vi "extract_carriers.vi"(0 "Carrier amplitudes":T14 format="%#_3p", 2 "Config":T15={"IO params"={"Conversion"={"Rate"=4.0, "Num cards"=2, "Out channels"=4}, "Carriers"={"Phase shift"=180.0, "Levels"=[[0.8, 0.8, 0.8], [0.03, 0.03, 0.03]], "Delay samples"=73.15}, "TCP"={"Host"="192.168.1.15", "Port"=6666, "Buffering"=6, "Timeout"=6}, "Input channel sign"=[1, 1, 1]}, "High rate STFT"={"Win param"=101.5, "Window type"=61, "Win order"=2, "DFT size"=64, "Channels"=[7], "Oversample"=64}, "Low rate STFT"={"Win param"=120.0, "Window type"=61, "Win order"=8, "DFT size"=64, "Channels"=[7], "Oversample"=64}, "Filtering "=[]} {"Filtering"."Distortion"."Limit" format="%#_3p"; "Filtering"."Distortion"."LF cut" format="%#_3p"; "Filtering"."Kalman"."Measure noise" format="%#_3p"; "Filtering"."Kalman"."Process noise" format="%#_3p"; "Filtering"."Hum"."Limit" format="%#_3p"; "Filtering"."Hum"."Frequency" format="%#_4p"; "Low rate STFT"."Oversample" min=1 step=1; "Low rate STFT"."Channels" min=0 step=1; "Low rate STFT"."DFT size" min=1 step=1; "Low rate STFT"."Window type" items=["Rectangle"=0, "Hanning"=1, "Hamming"=2, "Blackman-Harris"=3, "Exact Blackman"=4, "Blackman"=5, "Flat Top"=6, "4 Term B-Harris "=7, "7 Term B-Harris"=8, "Low Sidelobe"=9, "Blackman Nuttall"=11, "Triangle"=30, "Bartlett-Hanning"=31, "Bohman"=32, "Parzen"=33, "Welch"=34, "Kaiser"=60, "Dolph-Chebyshev"=61, "Gaussian"=62]; "High rate STFT"."Oversample" min=1 step=1; "High rate STFT"."Channels" min=0 step=1; "High rate STFT"."DFT size" min=1 step=1; "High rate STFT"."Window type" items=["Rectangle"=0, "Hanning"=1, "Hamming"=2, "Blackman-Harris"=3, "Exact Blackman"=4, "Blackman"=5, "Flat Top"=6, "4 Term B-Harris "=7, "7 Term B-Harris"=8, "Low Sidelobe"=9, "Blackman Nuttall"=11, "Triangle"=30, "Bartlett-Hanning"=31, "Bohman"=32, "Parzen"=33, "Welch"=34, "Kaiser"=60, "Dolph-Chebyshev"=61, "Gaussian"=62]; "IO params"."Input channel sign" min=-1 max=1 step=1; "IO params"."Carriers"."Levels" min=0.0 step=0.1; "IO params"."Conversion"."Rate" format="%#_8g"}, 3 "Modulation info":T21={"Fs full"=0.0, "Fs high"=0.0, "Fs low"=0.0, "Read size"=0, "FFT size low"=5000, "df low"=5000.0, "High carriers"=[], "Low carriers"=[], "Hi channels at low"=[7]} {"Hi channels at low" min=0 step=1; "Low carriers" format="%#_6p"; "High carriers" format="%#_6p"}, 4 "Demodulated signal":T1 format="%#_3p", 5 "Ref carrier amplitudes":T14 format="%#_3p", 7 "Display options":T2={"Display card"=0, "Signal"=enum."Raw data", "Source axis"=enum."X", "Sensor axis"=enum."X", "Spectrum parameters"={"Window"=enum."7 Term B-Harris", "FFT blocking"=enum."1", "Averaging"=5.0, "Order"=2}, "AC/DC"=FALSE, "Amplitude/Phase"=FALSE, "Levels selectors"=[], "Map selector"=enum."fire", "Restart Averaging"=FALSE, "Noise ref"=FALSE} {"Spectrum parameters"."Order" min=1 max=100; "Spectrum parameters"."Averaging" min=0.0 max=1000.0 step=1.0}, 8 "Level selector":T6, 9 "Spectrum":waveform(cdb)[](array[waveform]), 10 "Trace info":T11, 11 "Noise floor":dbl[][](array[numeric]) format="%#_6p") -> (14 "Levels":dbl[][](array[numeric]) format="%.3f")   [LabVIEW 2026]
uses:
  processing/modulation_info.ctl
  processing/ilemt_config.ctl
  system/IO_params.ctl
  processing/stft_params.ctl
  <vilib>/Analysis/4window.llb/windowTd.ctl
  processing/filter_params.ctl
  processing/detrend_mode.ctl
  processing/carrier_amplitudes.ctl
  levels_selector.ctl
  Level selector 1.ctl
  Level selector 4.ctl
  Level selector 3.ctl
  Level selector 2.ctl
  trace_info.ctl
  trace_channel.ctl
  main/ilemt_status.ctl
  display_options.ctl
  display_source.ctl
  axis_name.ctl
  spectrum_parameters.ctl
  processing/card_high_carrier_amplitudes.ctl
  processing/coupling_matrix.ctl
  <vilib>/Analysis/NI_AALPro.lvlib
panel:
  # "This VI generates user-friendly output arrays for the carrier levels and noise floor display."
  # "Complex demodulated signal, from get_display_data.  This is used to implement the \"Trace display\" source."
  # "High"
  # "Low"
  # "X"
  # "Y"
  # "Z"
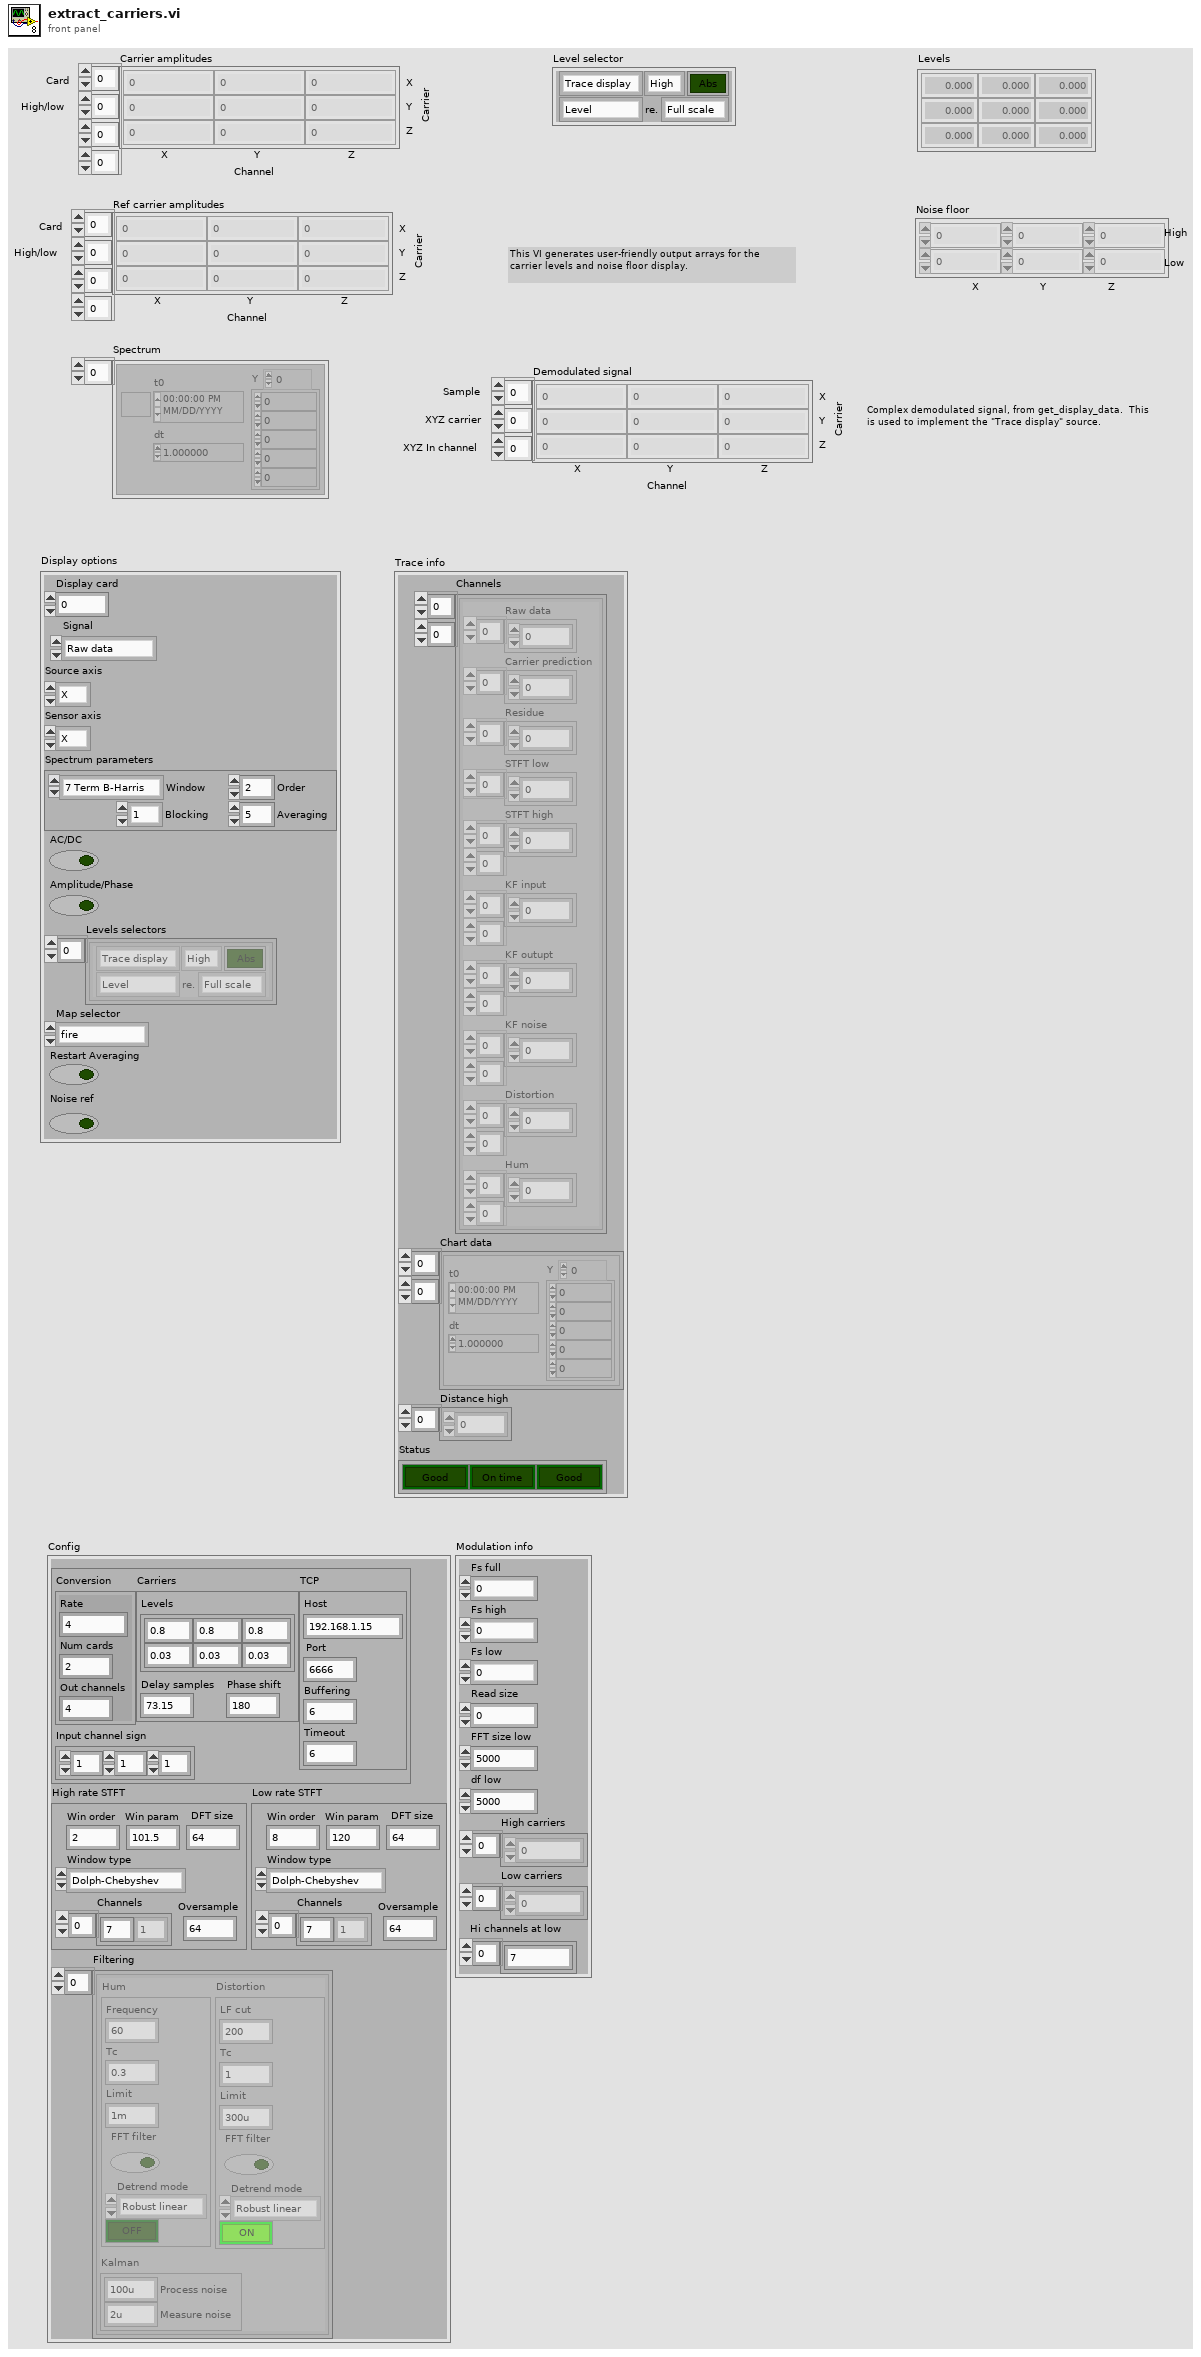
[diagram p1: front panel]
types:
  T1 = typedef "card_high_carrier_amplitudes.ctl" = cdb[][][]
  T2 = typedef "display_options.ctl" = cluster{"Display card":i32, "Signal":T3, "Source axis":T4, "Sensor axis":T4, "Spectrum parameters":T5, "AC/DC":bool, "Amplitude/Phase":bool, "Levels selectors":T6[], "Map selector":enum16{"fire", "rainbow", "grey", "inverse grey", "ice", "original"}, "Restart Averaging":bool, "Noise ref":bool}
  T3 = typedef "display_source.ctl" = enum16{"Raw data", "Carrier predict", "Residue", "STFT low", "STFT high", "KF input", "KF output", "KF noise", "Distortion", "Hum", "Distance high", "Chart high", "Chart low"}
  T4 = typedef "axis_name.ctl" = enum16{"X", "Y", "Z"}
  T5 = typedef "spectrum_parameters.ctl" = cluster{"Window":enum16{"None ", "Hanning", "Hamming", "Blackman-Harris", "Exact Blackman", "Blackman", "Flat Top", "4 Term B-Harris ", "7 Term B-Harris", "Low Sidelobe"}, "FFT blocking":enum16{"1", "2", "4", "8"}, "Averaging":dbl, "Order":u32}
  T6 = typedef "levels_selector.ctl" = cluster{"Signal source":T7, "Mode":T8, "re.":T9, "High/low":T10, "Sense":bool}
  T7 = typedef "Level selector 1.ctl" = enum16{"Trace display", "Carrier levels", "Ref levels"}
  T8 = typedef "Level selector 4.ctl" = enum16{"Level", "dB", "Phase", "Mismatch"}
  T9 = typedef "Level selector 3.ctl" = enum16{"Full scale", "Carrier", "Ref level", "Noise"}
  T10 = typedef "Level selector 2.ctl" = enum16{"High", "Low"}
  T11 = typedef "trace_info.ctl" = cluster{"Channels":T12[][], "Chart data":waveform(dbl)[][], "Distance high":dbl[], "Status":T13}
  T12 = typedef "trace_channel.ctl" = cluster{"Raw data":dbl[], "Carrier prediction":dbl[], "Residue":dbl[], "STFT low":cdb[], "STFT high":cdb[][], "KF input":cdb[][], "KF outupt":cdb[][], "KF noise":dbl[][], "Distortion":cdb[][], "Hum":cdb[][]}
  T13 = typedef "ilemt_status.ctl" = cluster{"NaN":bool, "Backlog":bool, "Clipping":bool}
  T14 = typedef "carrier_amplitudes.ctl" = cdb[][][][]
  T15 = typedef "ilemt_config.ctl" = cluster{"IO params":T16, "High rate STFT":T17, "Low rate STFT":T17, "Filtering ":T19[]}
  T16 = typedef "IO_params.ctl" = cluster{"Conversion":cluster{"Rate":dbl, "Num cards":u32, "Out channels":u32}, "Carriers":cluster{"Phase shift":dbl, "Levels":dbl[][], "Delay samples":dbl}, "TCP":cluster{"Host":string, "Port":i32, "Buffering":u32, "Timeout":u32}, "Input channel sign":i32[]}
  T17 = typedef "stft_params.ctl" = cluster{"Win param":dbl, "Window type":T18, "Win order":i32, "DFT size":i32, "Channels":i32[], "Oversample":i32}
  T18 = typedef "NI_AALPro.lvlib/windowTd.ctl" = u32
  T19 = typedef "filter_params.ctl" = cluster{"Hum":cluster{"Frequency":dbl, "Tc":dbl, "Limit":dbl, "FFT filter":bool, "Detrend mode":T20, "Enable":bool}, "Kalman":cluster{"Process noise":dbl, "Measure noise":dbl}, "Distortion":cluster{"LF cut":dbl, "Tc":dbl, "Limit":dbl, "FFT filter":bool, "Detrend mode":T20, "Enable":bool}}
  T20 = typedef "detrend_mode.ctl" = enum16{"Zero mean", "Linear", "Robust linear"}
  T21 = typedef "modulation_info.ctl" = cluster{"Fs full":dbl, "Fs high":dbl, "Fs low":dbl, "Read size":i32, "FFT size low":i32, "df low":dbl, "High carriers":dbl[], "Low carriers":dbl[], "Hi channels at low":i32[]}
  T22 = typedef "coupling_matrix.ctl" = cdb[][]
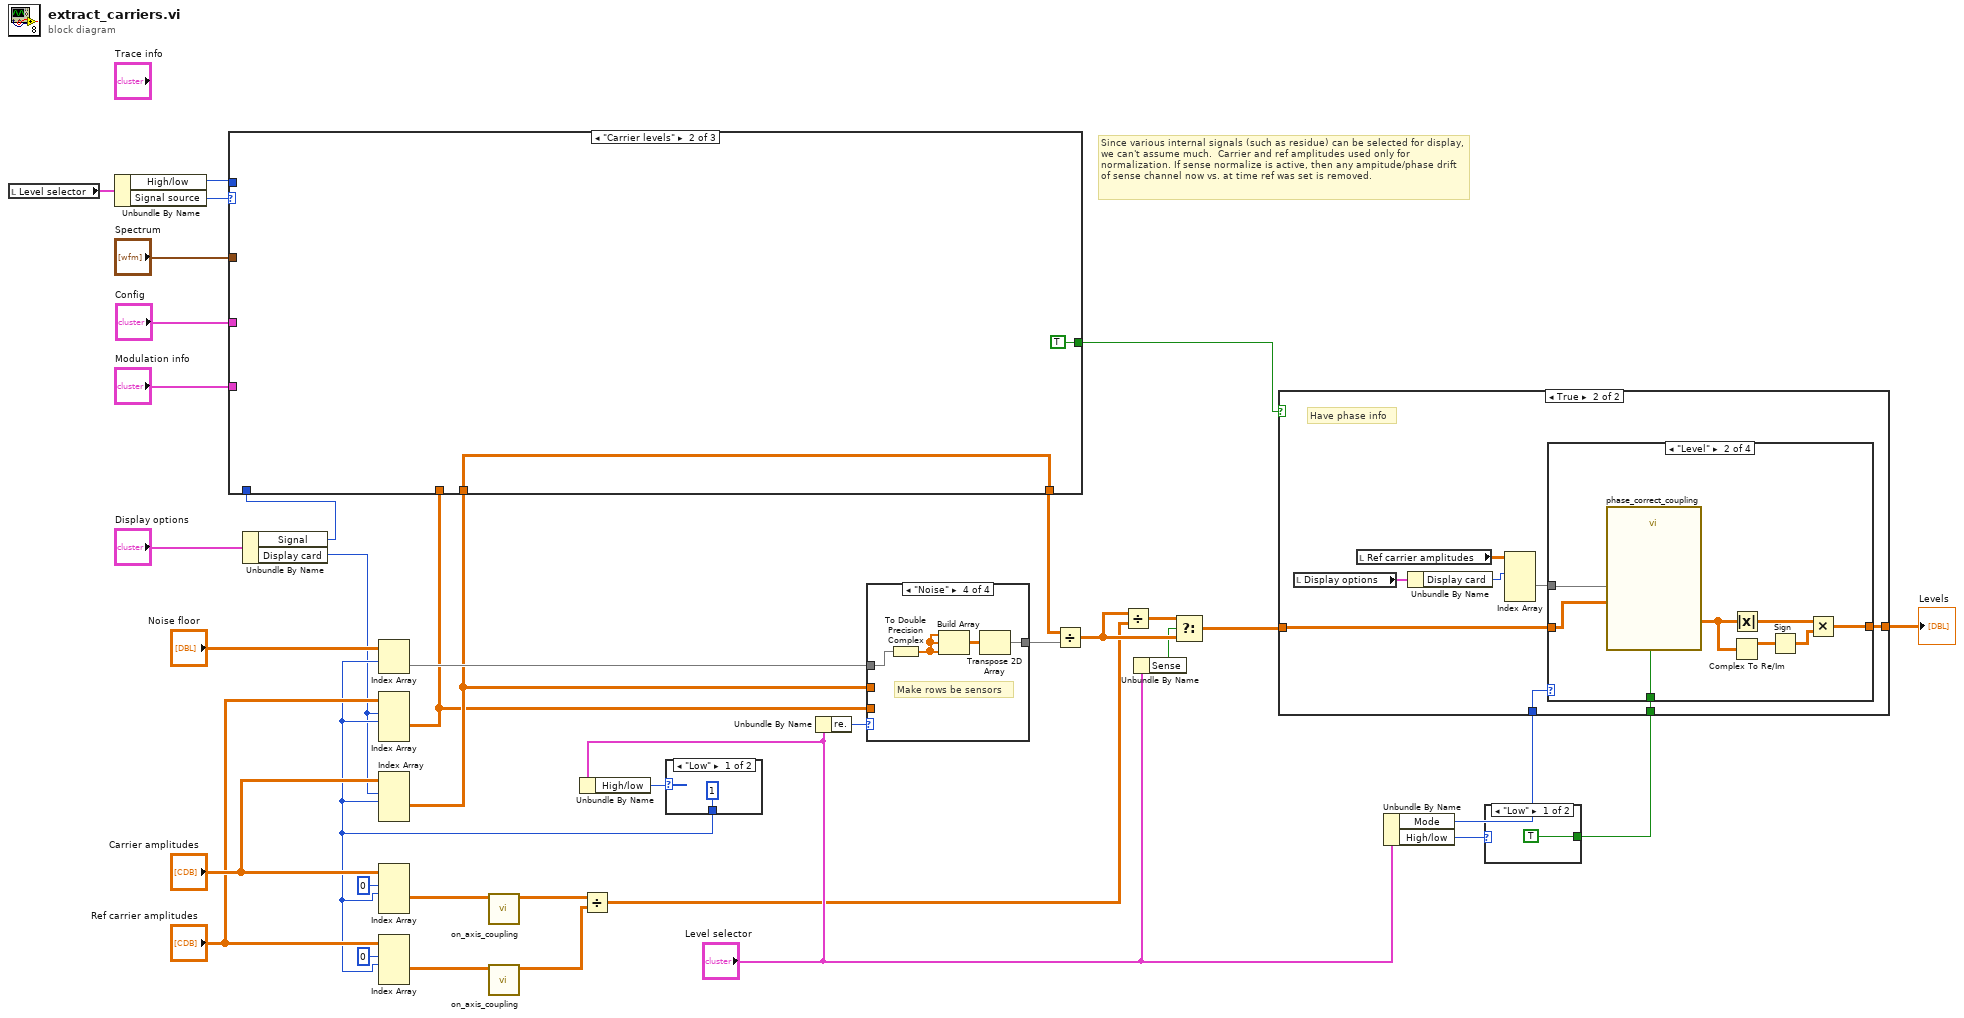
[diagram p0: block diagram]
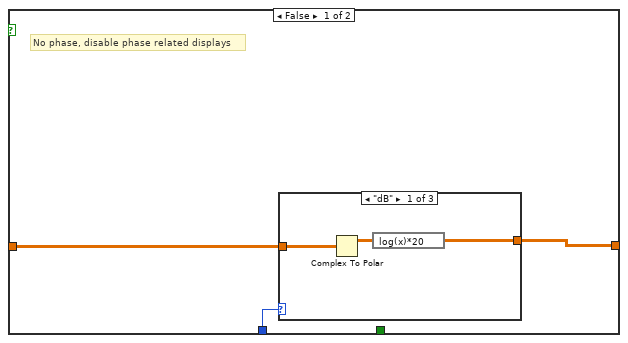
[diagram p2: hidden frame]
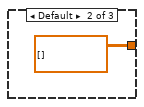
[diagram p3: hidden frame]
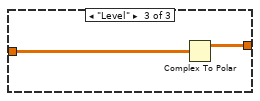
[diagram p4: hidden frame]
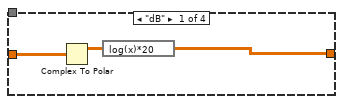
[diagram p5: hidden frame]
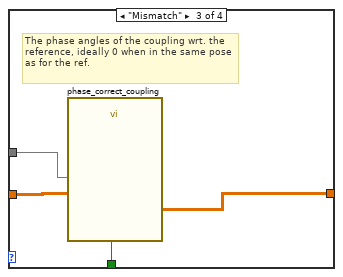
[diagram p6: hidden frame]
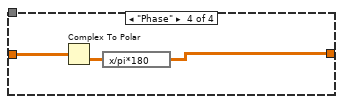
[diagram p7: hidden frame]
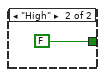
[diagram p8: hidden frame]
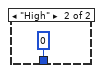
[diagram p9: hidden frame]
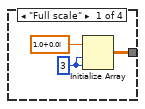
[diagram p10: hidden frame]
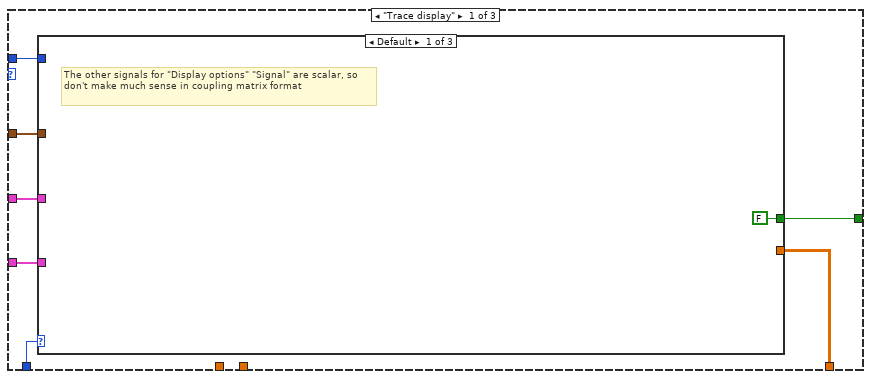
[diagram p13: hidden frame]
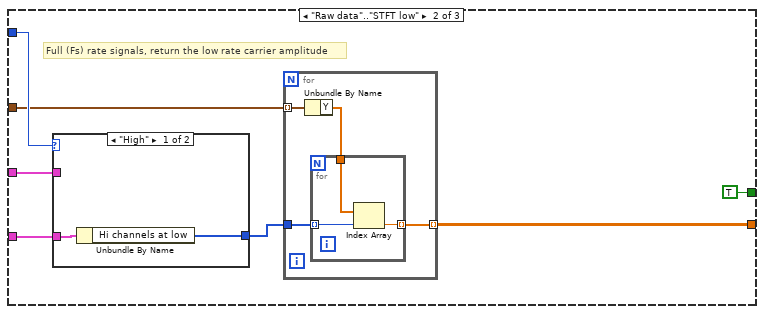
[diagram p14: hidden frame]
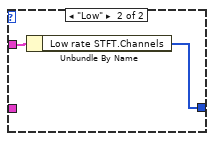
[diagram p15: hidden frame]
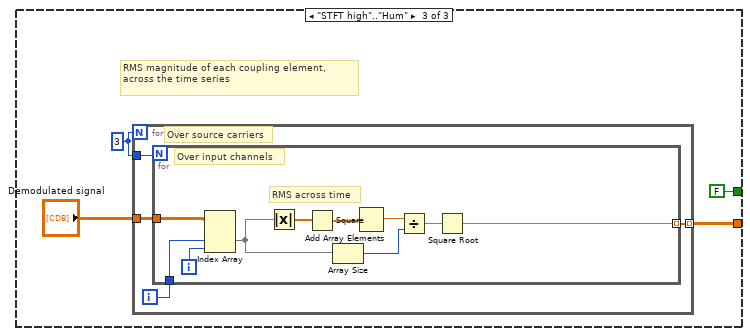
[diagram p16: hidden frame]
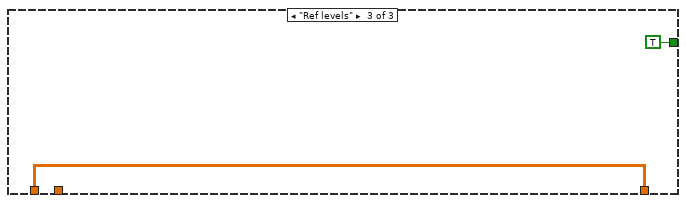
[diagram p17: hidden frame]
diagram:
  # "Since various internal signals (such as residue) can be selected for display, we can't assume much.  Carrier and ref amplitudes used only for normalization. If sense normalize is active, then any ampitude/phase drift of sense channel now vs. at time ref was set is removed."
  n1 = local read "Level selector"() -> (w25:T6)
  n2 = Unbundle By Name(w25) -> ("High/low"=w36:T10, "Signal source"=w37:T7)
  n3 = Unbundle By Name("Display options") -> ("Signal"=w7:T3, "Display card"=w3:i32)
  n4 = Unbundle By Name("Level selector") -> ("High/low"=w34:T10)
  n5 = case shown="\"Low\"" w34 {
    tunnel: [1 0] -> w11
    frame "Low" {
    }
    frame "High" {
    }
  }
  n6 = Index Array(array="Noise floor", index (row)=w11) -> (element=w23:dbl[])  [unwired: 1 in]
  n7 = Index Array(array="Ref carrier amplitudes", index (dim 0)=w3, index (dim 1)=w11) -> (element=w21:cdb[][])  [unwired: 2 in]
  n8 = Index Array(array="Carrier amplitudes", index (dim 0)=w3, index (dim 1)=w11) -> (element=w22:cdb[][])  [unwired: 2 in]
  n9 = case shown="\"Carrier levels\"" w37 {
    tunnel: [w45 w85 w87] -> w33
    tunnel: w36 -> [w46 _ _]
    tunnel: w22 -> [_ w85 _]
    tunnel: w21 -> [_ _ w87]
    tunnel: w7 -> [w44 _ _]
    tunnel: "Modulation info" -> [w43 _ _]
    tunnel: "Spectrum" -> [w42 _ _]
    tunnel: "Config" -> [w41 _ _]
    tunnel: [w40 TRUE TRUE] -> w1
    frame "Trace display" {
      n10 = case shown="Default" w44 {
        tunnel: w46 -> [_ w54 _]
        tunnel: [_ w53 w69] -> w45
        tunnel: w43 -> [_ w51 _]
        tunnel: w42 -> [_ w50 _]
        tunnel: w41 -> [_ w49 _]
        tunnel: [FALSE TRUE FALSE] -> w40
        frame Default {
          # "The other signals for \"Display options\" \"Signal\" are scalar, so don't make much sense in coupling matrix format"
        }
        frame "Raw data".."STFT low" {
          # "Full (Fs) rate signals, return the low rate carrier amplitude"
          n11 = case shown="\"High\"" w54 {
            tunnel: [w62 w64] -> w52
            tunnel: w49 -> [_ w65]
            tunnel: w51 -> [w63 _]
            frame "High" {
              n12 = Unbundle By Name(w63) -> ("Hi channels at low"=w62:i32[])
            }
            frame "Low" {
              n13 = Unbundle By Name(w65) -> ("Low rate STFT.Channels"=w64:i32[])
            }
          }
          n14 = for {
            tunnel: w50 -> [w56] mode=indexing
            tunnel: w52 -> [w58]
            tunnel: [w57] -> w53 mode=indexing
            n15 = Unbundle By Name(w56) -> ("Y"=w55:cdb[])
            n16 = for {
              tunnel: w58 -> [w59] mode=indexing
              tunnel: w55 -> [w61]
              tunnel: [w60] -> w57 mode=indexing
              n17 = Index Array(array=w61, index=w59) -> (element=w60:cdb)
            }
          }
        }
        frame "STFT high".."Hum" {
          w67 = 3
          # "RMS magnitude of each coupling element, across the time series"
          n18 = for {
            N: w67 -> [_]
            tunnel: "Demodulated signal" -> [w73]
            tunnel: [w72] -> w69 mode=indexing
            tunnel: w67 -> [w71]
            i -> [w70]
            # "Over source carriers"
            n19 = for {
              N: w71 -> [_]
              tunnel: w73 -> [w79]
              tunnel: [w74] -> w72 mode=indexing
              tunnel: w70 -> [w77]
              i -> [w78]
              # "RMS across time"
              # "Over input channels"
              n20 = Index Array(array=w79, index (dim 1)=w77, index (dim 2)=w78) -> (element=w76:cdb[])  [unwired: 1 in]
              n21 = Absolute Value(x=w76) -> (abs(x)=w80:dbl[])
              n22 = Square(x=w80) -> (x^2=w83:dbl[])
              n23 = Array Size(array=w76) -> (size(s)=w81:i32)
              n24 = Add Array Elements(numeric array=w83) -> (sum=w82:dbl)
              n25 = Divide(x=w82, y=w81) -> (x/y=w75:dbl)
              n26 = Square Root(x=w75) -> (sqrt(x)=w74:dbl)
            }
          }
        }
      }
    }
    frame "Carrier levels" {
    }
    frame "Ref levels" {
    }
  }
  n27 = Index Array(array="Carrier amplitudes", index (dim 0)=0 ("index (vol)"), index (dim 1)=w11) -> (element=w9:cdb[][])  [unwired: 2 in]
  n28 = Index Array(array="Ref carrier amplitudes", index (dim 0)=0 ("index (vol)"), index (dim 1)=w11) -> (element=w10:cdb[][])  [unwired: 2 in]
  n29 = call "on_axis_coupling.vi"("Sense coupling"=w9) -> ("Sense amplitudes"=w20:T22)  [unwired: 10 in]
  n30 = call "on_axis_coupling.vi"("Sense coupling"=w10) -> ("Sense amplitudes"=w19:T22)  [unwired: 10 in]
  n31 = Divide(x=w20, y=w19) -> (x/y=w8:T22)
  n32 = Unbundle By Name("Level selector") -> ("re."=w35:T9)
  n33 = case shown="\"Noise\"" w35 {
    tunnel: w22 -> [_ w91 _ _]
    tunnel: [w88 w91 w92 w93] -> w32
    tunnel: w21 -> [_ _ w92 _]
    tunnel: w23 -> [_ _ _ w96]
    frame "Full scale" {
      w89 = 3 ("dimension size")
      n34 = Initialize Array(cdb 1.0+0.0i, w89, w89) -> (w88:cdb[][])
    }
    frame "Carrier" {
    }
    frame "Ref level" {
    }
    frame "Noise" {
      # "Make rows be sensors"
      n35 = To Double Precision Complex(1:w96) -> (0:w95:cdb[])
      n36 = Build Array(w95, w95, w95) -> (w94:cdb[][])
      n37 = Transpose 2D Array(2D array=w94) -> (transposed array=w93:cdb[][])
    }
  }
  n38 = Divide(x=w33, y=w32) -> (x/y=w30:cdb[][])
  n39 = Divide(x=w30, y=w8) -> (x/y=w31:T22)
  n40 = Unbundle By Name("Level selector") -> ("Sense"=w18:bool)
  n41 = Select(t=w31, s=w18, f=w30) -> (s? t:f=w17:T22)
  n42 = Unbundle By Name("Level selector") -> ("Mode"=w29:T8, "High/low"=w27:T10)
  n43 = case shown="\"Low\"" w27 {
    tunnel: [TRUE FALSE] -> w26
    frame "Low" {
    }
    frame "High" {
    }
  }
  n44 = case shown="True" w1 {
    tunnel: w29 -> [w101 w115]
    tunnel: [w99 w114] -> w28
    tunnel: w26 -> [_ w113]
    tunnel: w17 -> [w100 w112]
    frame False {
      # "No phase, disable phase related displays"
      n45 = case shown="\"dB\"" w101 {
        tunnel: w100 -> [w104 _ w106]
        tunnel: [w102 T22 [] ("Sense amplitudes") w107] -> w99
        frame "dB" {
          n46 = Complex To Polar(r * e^(i*theta)=w104) -> (r=w103:dbl[][])  [unwired: 1 out]
          n47 = expression code="log(x)*20"(w103) -> (w102:dbl[][])
        }
        frame Default {
        }
        frame "Level" {
          n48 = Complex To Polar(r * e^(i*theta)=w106) -> (r=w107:dbl[][])  [unwired: 1 out]
        }
      }
    }
    frame True {
      # "Have phase info"
      n49 = local read "Display options"() -> (w109:T2)
      n50 = local read "Ref carrier amplitudes"() -> (w111:T14)
      n51 = Unbundle By Name(w109) -> ("Display card"=w108:i32)
      n52 = Index Array(array=w111, index (dim 0)=w108) -> (element=w110:cdb[][][])  [unwired: 3 in]
      n53 = case shown="\"Level\"" w115 {
        tunnel: w112 -> [w118 w124 w128 w132]
        tunnel: [w116 w121 w127 w131] -> w114
        tunnel: w110 -> [_ w126 w130 _]
        tunnel: w113 -> [_ w125 w129 _]
        frame "dB" {
          n54 = Complex To Polar(r * e^(i*theta)=w118) -> (r=w117:dbl[][])  [unwired: 1 out]
          n55 = expression code="log(x)*20"(w117) -> (w116:dbl[][])
        }
        frame "Level" {
          n56 = call "phase_correct_coupling.vi"("Is low?"=w125, "Complex coupling"=w124, "Ref carrier ampl"=w126) -> ("Phase corrected coupling"=w120:cdb[][])  [unwired: 7 in, 1 out]
          n57 = Absolute Value(x=w120) -> (abs(x)=w123:dbl[][])
          n58 = Complex To Re/Im(x + iy=w120) -> (x=w119:dbl[][])  [unwired: 1 out]
          n59 = Sign(1:w119) -> (0:w122:dbl[][])
          n60 = Multiply(x=w123, y=w122) -> (x*y=w121:dbl[][])
        }
        frame "Mismatch" {
          # "The phase angles of the coupling wrt. the reference, ideally 0 when in the same pose as for the ref."
          n61 = call "phase_correct_coupling.vi"("Is low?"=w129, "Complex coupling"=w128, "Ref carrier ampl"=w130) -> ("Phase mismatch"=w127:dbl[][])  [unwired: 7 in, 1 out]
        }
        frame "Phase" {
          n62 = Complex To Polar(r * e^(i*theta)=w132) -> (theta=w133:dbl[][])  [unwired: 1 out]
          n63 = expression code="x/pi*180"(w133) -> (w131:dbl[][])
        }
      }
    }
  }
  "Levels" <- w28
